vi "reserveDevice.vi"(8 "error in (no error)":errorcluster, 10 "deviceName":string, 11 "HWController in":refnum<class "HWController.lvclass">) -> (0 "error out":errorcluster, 3 "HWController out":refnum<class "HWController.lvclass">)   [LabVIEW 2009, in "Hardware.lvlib" / "HWControllers.lvlib" / "HWController.lvclass"]
doc: "Reserve the HW so no one else can use it"
uses:
  HWController.lvclass
  HWController.lvclass/HWController.ctl
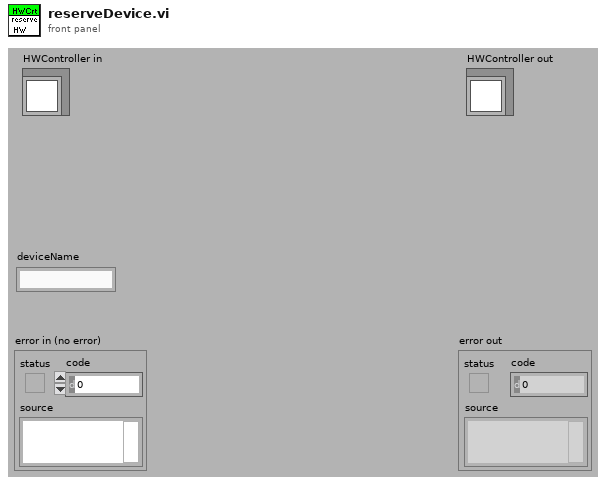
[diagram p1: front panel]
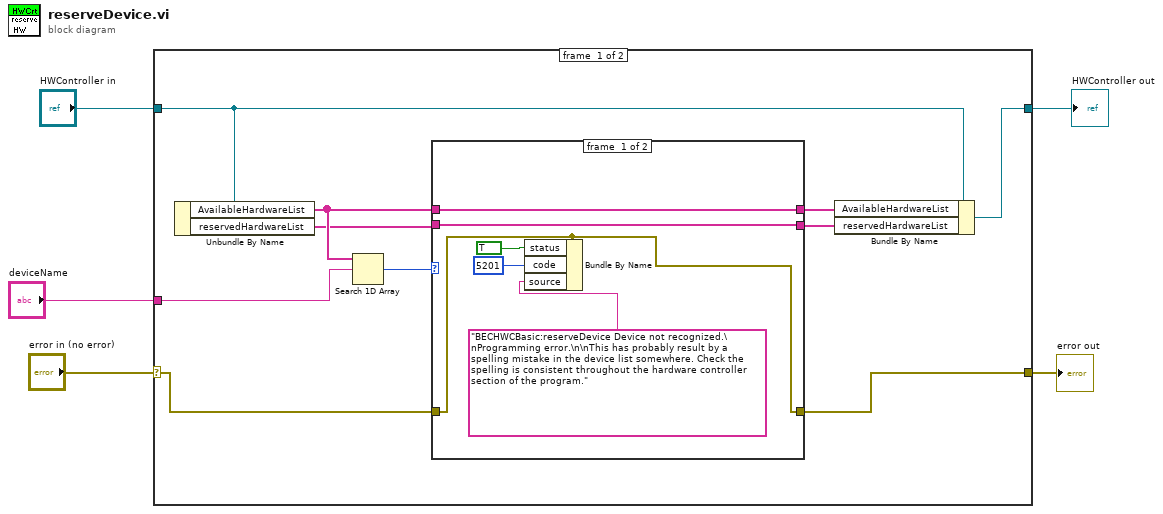
[diagram p0: block diagram]
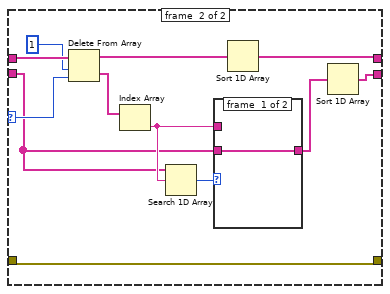
[diagram p2: hidden frame]
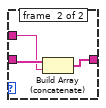
[diagram p3: hidden frame]
diagram:
  n1 = case shown="No Error" "error in (no error)" {
    selector: "error in (no error)" -> [w13 w39]
    tunnel: [w12 w39] -> w4
    tunnel: [w6 w38] -> w1
    tunnel: "HWController in" -> [w7 w38]
    tunnel: "deviceName" -> [w15 _]
    frame #0 {
      n2 = Unbundle By Name(w7) -> ("AvailableHardwareList"=w11:string[], "reservedHardwareList"=w8:string[])
      n3 = Search 1D Array(1D array=w11, element=w15) -> (index of element=w14:i32)  [unwired: 1 in]
      n4 = case shown="-1" w14 {
        selector: w14 -> [_ w31]
        tunnel: w13 -> [w16 w33]
        tunnel: [w16 w33] -> w12
        tunnel: w11 -> [w18 w32]
        tunnel: [w18 w25] -> w10
        tunnel: [w17 w23] -> w9
        tunnel: w8 -> [w17 w26]
        frame #0 {
          n5 = Bundle By Name(cluster=w16, "status"=TRUE, "code"=5201, "source"="BECHWCBasic:reserveDevice Device not recognized.\nProgramming error.\n\nThis has probably result by a spelling mistake in the device list somewhere. Check the spelling is consistent throughout the hardware controller section of the program.") -> ()  [unwired: 1 out]
        }
        frame #1 {
          n6 = Delete From Array(array=w32, length=1, index=w31) -> (deleted portion=w29:string[], array with subset deleted=w24:string[])
          n7 = Index Array(array=w29) -> (element=w27:string)  [unwired: 1 in]
          n8 = Search 1D Array(1D array=w26, element=w27) -> (index of element=w28:i32)  [unwired: 1 in]
          n9 = case shown="-1" w28 {
            tunnel: w27 -> [_ w36]
            tunnel: w26 -> [w34 w37]
            tunnel: [w34 w35] -> w22
            frame #0 {
            }
            frame #1 {
              n10 = Build Array (concatenate)(w37, w36) -> (w35:string[])
            }
          }
          n11 = Sort 1D Array(array=w24) -> (sorted array=w25:string[])
          n12 = Sort 1D Array(array=w22) -> (sorted array=w23:string[])
        }
      }
      n13 = Bundle By Name(cluster=w7, "AvailableHardwareList"=w10, "reservedHardwareList"=w9) -> (w6:refnum<class "HWController.lvclass">)
    }
    frame #1 {
    }
  }
  "error out" <- w4
  "HWController out" <- w1
